vi "subPanel - Read Value.vi"(8 "Error In":errorcluster, 10 "subPanel Ref":refnum<vi>, 11 "CtlRef":refnum<vi>) -> (0 "Error Out":errorcluster, 1 "Pnl CtlRef":refnum<vi>, 2 "Pnl Controls[]":refnum<vi>[](array[refnum]), 3 "CtlRef":refnum<vi>)   [LabVIEW 2013]
panel:
  in  "ComboBox":refnum<vi>
  in  "Combobox":refnum<vi>
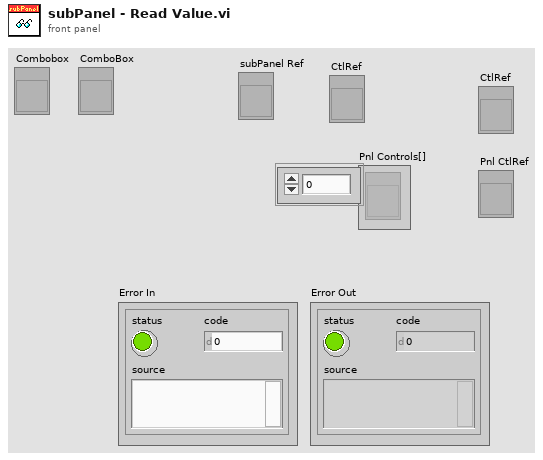
[diagram p1: front panel]
types:
  T1 = typedef "LVComboBoxStrsAndValuesArrayTypeDef.ctl" = cluster{"String":string, "Value":string}[]
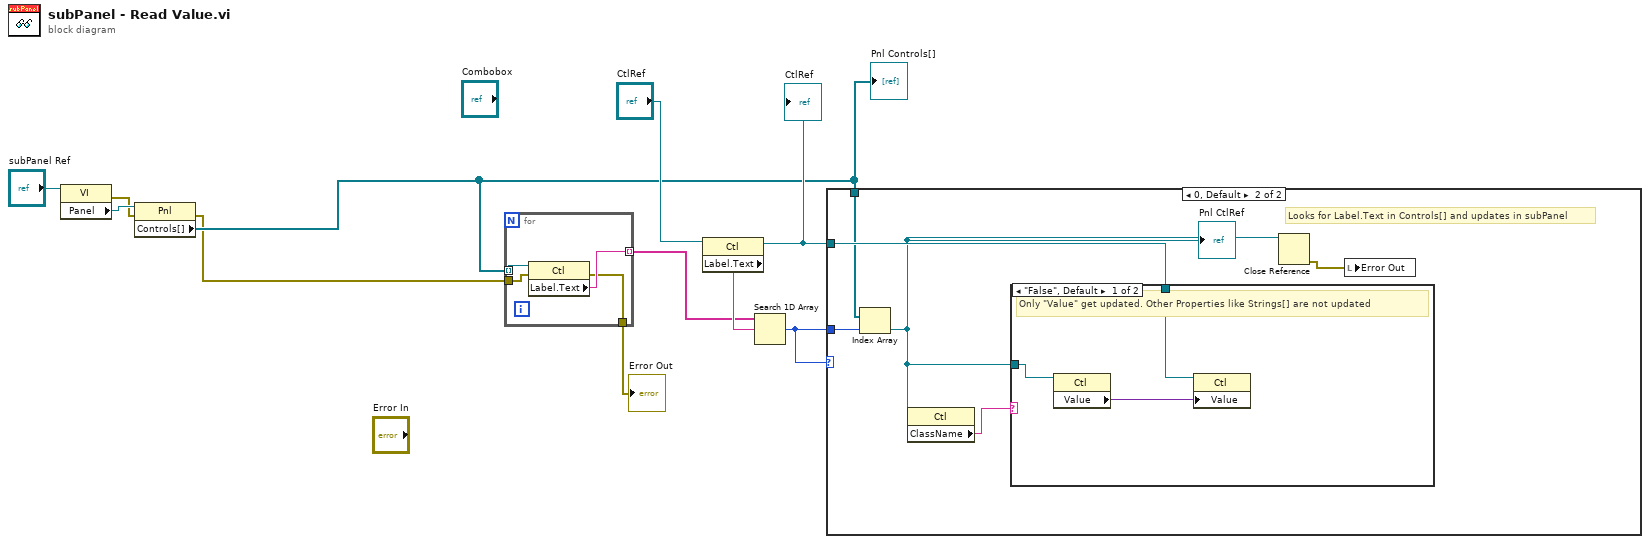
[diagram p0: block diagram]
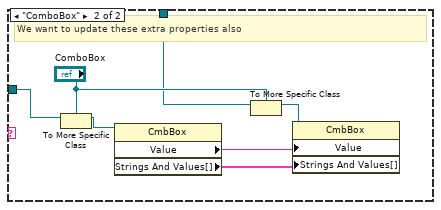
[diagram p3: hidden frame]
diagram:
  n1 = property class="VI"(reference="subPanel Ref") -> (error out=w4:errorcluster, "Panel"=w7:refnum<vi>)  [unwired: 1 in, 1 out]
  n2 = property class="Pnl"(reference=w7, error in=w4) -> (error out=w3:errorcluster, "Controls[]"=w5:refnum<vi>[])  [unwired: 1 out]
  "Pnl Controls[]" <- w5
  n3 = for {
    tunnel: w5 -> [w15] mode=indexing
    tunnel: [w14] -> w9 mode=indexing
    tunnel: w3 -> [w13]
    tunnel: [w12] -> w2
    n4 = property class="Ctl"(reference=w15, error in=w13) -> (error out=w12:errorcluster, "Label.Text"=w14:string)  [unwired: 1 out]
  }
  "Error Out" <- w2
  n5 = property class="Ctl"(reference="CtlRef") -> (reference out=w8:refnum<vi>, "Label.Text"=w10:string)  [unwired: 1 in, 1 out]
  "CtlRef" <- w8
  n6 = Search 1D Array(1D array=w9, element=w10) -> (index of element=w1:i32)  [unwired: 1 in]
  n7 = case shown="0, Default" w1 {
    tunnel: w1 -> [_ w21]
    tunnel: w8 -> [_ w19]
    tunnel: w5 -> [_ w18]
    frame -1 {
    }
    frame 0, Default {
      # "Looks for Label.Text in Controls[] and updates in subPanel"
      n8 = Index Array(array=w18, index=w21) -> (element=w16:refnum<vi>)
      "Pnl CtlRef" <- w16
      n9 = property class="Ctl"(reference=w16) -> ("ClassName"=w20:string)  [unwired: 1 in, 2 out]
      n10 = case shown="\"False\", Default" w20 {
        tunnel: w16 -> [w22 w31]
        tunnel: w19 -> [w24 w25]
        frame "False", Default {
          # "Only \"Value\" get updated. Other Properties like Strings[] are not updated"
          n11 = property class="Ctl"(reference=w22) -> ("Value"=w23:variant)  [unwired: 1 in, 2 out]
          n12 = property class="Ctl"(reference=w24, "Value"=w23) -> ()  [unwired: 1 in, 2 out]
        }
        frame "ComboBox" {
          # "We want to update these extra properties also"
          n13 = To More Specific Class(target class="ComboBox", reference=w31) -> (specific class reference=w30:refnum<vi>)  [unwired: 1 in, 1 out]
          n14 = property class="CmbBox"(reference=w30) -> ("Value"=w27:string, "Strings And Values[]"=w26:T1)  [unwired: 1 in, 2 out]
          n15 = To More Specific Class(target class="ComboBox", reference=w25) -> (specific class reference=w28:refnum<vi>)  [unwired: 1 in, 1 out]
          n16 = property class="CmbBox"(reference=w28, "Value"=w27, "Strings And Values[]"=w26) -> ()  [unwired: 1 in, 2 out]
        }
      }
      n17 = Close Reference(reference=w16) -> (error out=w17:errorcluster)  [unwired: 1 in]
      n18 = local write "Error Out"(w17) -> ()
    }
  }
